vi "NML Assert Ren.vi"(8 "error in (no error)":errorcluster {"code" format="%.0x"}, 11 "VISA resource name":refnum<visa-resource-name>) -> (0 "error out":errorcluster {"code" format="%.0x"}, 3 "dup VISA Session":refnum<visa-resource-name>)   [LabVIEW 2019]
uses:
  <vilib>/Instr/_visa.llb/VISA GPIB Control REN Mode.ctl
panel:
  out "Interface Information:Interface Type":u16(ring)=1 items=["GPIB"=1, "VXI"=2, "GPIB-VXI"=3, "Serial"=4, "PXI"=5, "TCPIP"=6, "USB"=7, "FireWire"=9]
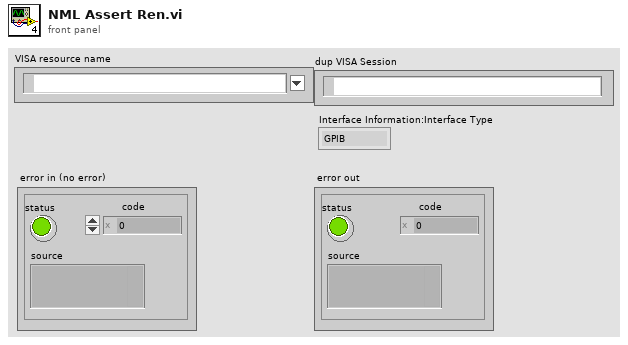
[diagram p1: front panel]
types:
  T1 = typedef "VISA GPIB Control REN Mode.ctl" = u16
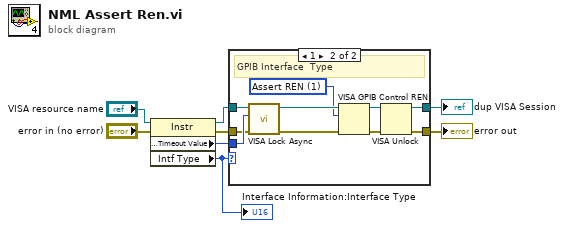
[diagram p0: block diagram]
diagram:
  n1 = property class="Instr"(reference="VISA resource name", error in="error in (no error)") -> (reference out=w6:refnum<visa-resource-name>, error out=w7:errorcluster, "General Settings:Timeout Value"=w8:u32, "Intf Type"=w1:u16)
  "Interface Information:Interface Type" <- w1
  n2 = case shown="1" w1 {
    tunnel: w8 -> [_ w20]
    tunnel: w7 -> [w9 w19]
    tunnel: w6 -> [w10 w18]
    tunnel: [w9 w17] -> w3
    tunnel: [w10 w16] -> w2
    frame Default {
    }
    frame 1 {
      w11 = T1 1 items=["Deassert REN", "Assert REN", "Go To Local; Deassert REN ", "Assert REN; Address Device", "Local Lockout (Addressed Devices)", "Local Lockout (This Device)", "Go To Local"] ("Mode")
      # "GPIB Interface  Type"
      n3 = call <vilib>:"VISA Lock Async.vi"("error in (no error)"=w19, "timeout (0)"=w20, "VISA resource name"=w18) -> ("error out"=w13:errorcluster, "VISA resource name out"=w12:refnum<visa-resource-name>)  [unwired: 6 in, 1 out]
      n4 = VISA GPIB Control REN(8:w13, 10:w11, 11:w12) -> (0:w15:errorcluster, 3:w14:refnum<visa-resource-name>)
      n5 = VISA Unlock(8:w15, 11:w14) -> (0:w17:errorcluster, 3:w16:refnum<visa-resource-name>)
    }
  }
  "error out" <- w3
  "dup VISA Session" <- w2
